vi "PathPlanner_PathFinder_TopKey.vi"(11 "Open":map{i32, T1}(c390)) -> (0 "Found":bool, 1 "DoublePair":T1, 3 "PathPlannerFinderGridPosition":T2)   [LabVIEW 2019]
uses:
  PathPlannerLib24/TypeDef/PathPlannerFinderDoublePair.ctl
  PathPlannerLib24/TypeDef/PathPlannerFinderGridPosition.ctl
  PathPlannerLib24/VI/PathPlanner_GridPosition_New.vi
  PathPlannerLib24/PathPlanner24.lvlib
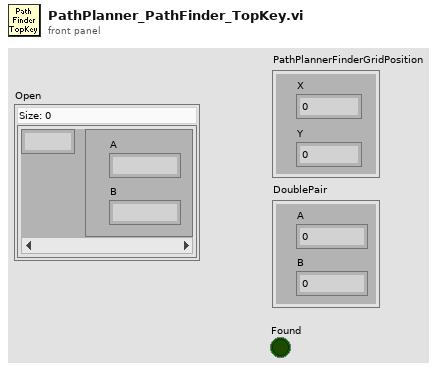
[diagram p1: front panel]
types:
  T1 = typedef "PathPlanner24.lvlib/PathPlannerFinderDoublePair.ctl" = cluster{"A":dbl, "B":dbl}
  T2 = typedef "PathPlanner24.lvlib/PathPlannerFinderGridPosition.ctl" = cluster{"X":i32, "Y":i32}
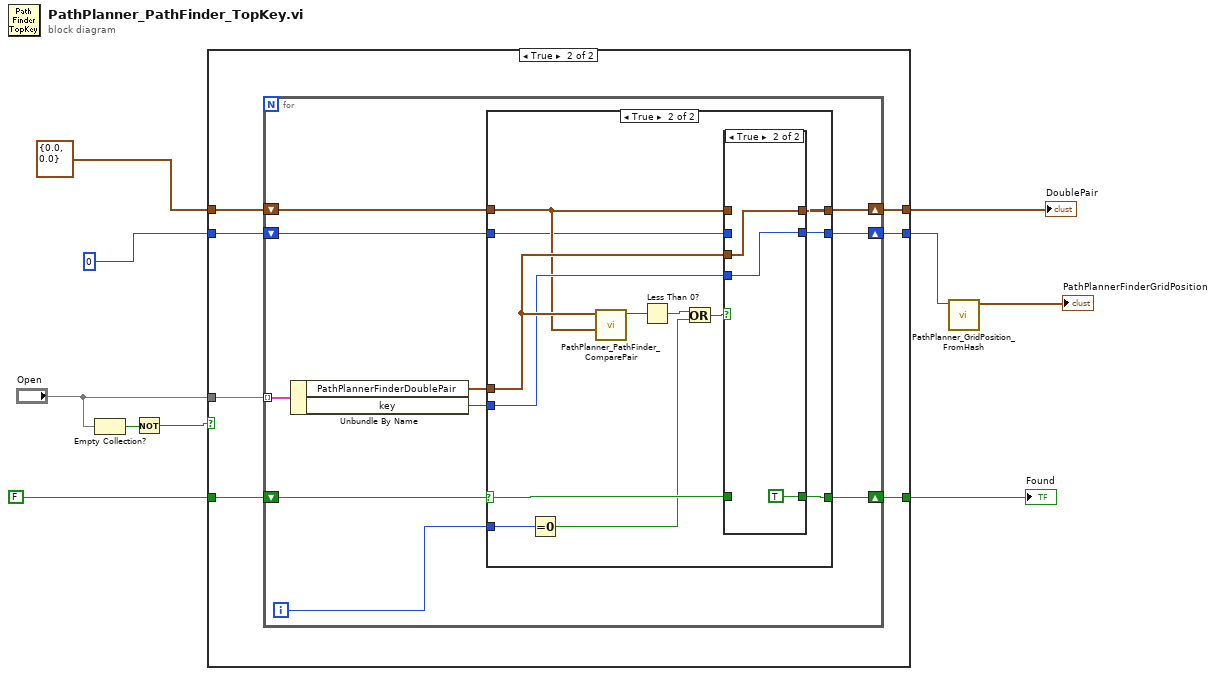
[diagram p0: block diagram]
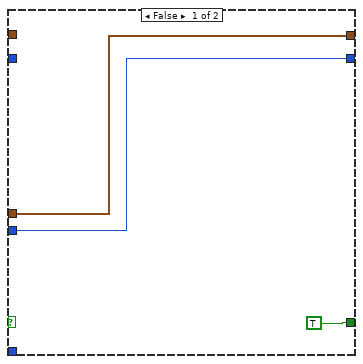
[diagram p3: hidden frame]
diagram:
  n1 = Empty Collection?(1:"Open") -> (0:w3:bool)
  n2 = Not(x=w3) -> (.not. x?=w2:bool)
  n3 = case shown="True" w2 {
    tunnel: FALSE -> [w11 w20]
    tunnel: [w11 w19] -> w9
    tunnel: T1 {"A"=0.0, "B"=0.0} ("DoublePair") -> [w13 w18]
    tunnel: [w13 w17] -> w8
    tunnel: 0 ("key") -> [w12 w16]
    tunnel: [w12 w15] -> w6
    tunnel: "Open" -> [_ w14]
    frame False {
    }
    frame True {
      n4 = for {
        tunnel: w14 -> [w29] mode=indexing
        shift-right: [w24] -> w19
        shift-left: w20 -> [w30]
        shift-right: [w28] -> w17
        shift-left: w18 -> [w23]
        shift-right: [w26] -> w15
        shift-left: w16 -> [w22]
        i -> [w21]
        n5 = Unbundle By Name(w29) -> ("PathPlannerFinderDoublePair"=w27:T1, "key"=w25:i32)
        n6 = case shown="True" w30 {
          selector: w30 -> [_ w38]
          tunnel: [w33 w45] -> w28
          tunnel: w27 -> [w33 w44]
          tunnel: [w32 w43] -> w26
          tunnel: w25 -> [w32 w42]
          tunnel: [TRUE w39] -> w24
          tunnel: w23 -> [_ w41]
          tunnel: w22 -> [_ w40]
          tunnel: w21 -> [_ w35]
          frame False {
          }
          frame True {
            n7 = Equal To 0?(x=w35) -> (x = 0?=w34:bool)
            n8 = call "PathPlanner_PathFinder_ComparePair.vi"("B"=w41, "A"=w44) -> ("Compare"=w46:i32)  [unwired: 9 in]
            n9 = Less Than 0?(x=w46) -> (x < 0?=w36:bool)
            n10 = Or(x=w36, y=w34) -> (x .or. y?=w37:bool)
            n11 = case shown="True" w37 {
              tunnel: [w49 w52] -> w45
              tunnel: w44 -> [_ w52]
              tunnel: [w48 w51] -> w43
              tunnel: w42 -> [_ w51]
              tunnel: w41 -> [w49 _]
              tunnel: w40 -> [w48 _]
              tunnel: [w47 TRUE] -> w39
              tunnel: w38 -> [w47 _]
              frame False {
              }
              frame True {
              }
            }
          }
        }
      }
    }
  }
  "DoublePair" <- w8
  "Found" <- w9
  n12 = call "PathPlanner_GridPosition_FromHash.vi"("Hash"=w6) -> ("GridPosition"=→"PathPlannerFinderGridPosition":T2)  [unwired: 10 in]
